vi "OA Set Int.vi"(9 "iIntValue":i32, 10 "pcModeParam":string, 11 "pcModeName":string) -> (3 "function return":u32)   [LabVIEW 2018, in "AndorSDK.lvlib"]
doc: "EXPNETTYPE unsigned int WINAPI OA_SetInt(const char * const pcModeName, const char * pcModeParam, const int iIntValue);"
uses:
  AndorSDK.lvlib
  ATMCD32D.dll
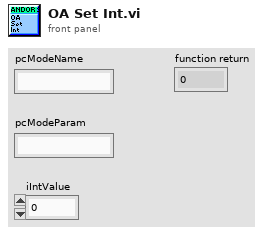
[diagram p1: front panel]
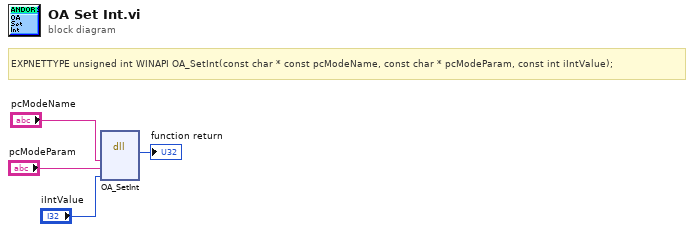
[diagram p0: block diagram]
diagram:
  # "EXPNETTYPE unsigned int WINAPI OA_SetInt(const char * const pcModeName, const char * pcModeParam, const int iIntValue);"
  n1 = dll-call lib="PTH2babs E\nPersönliches02 - Arbeit03-HiwijobsLabviewCodelibANDOR\tAndor SDK\nATMCD32D.*" fn="OA_SetInt"("pcModeName"="pcModeName", "pcModeParam"="pcModeParam", "iIntValue"="iIntValue") -> (→"function return":u32)  [unwired: 6 in, 2 out]
